vi "Configure DC Mode.vi"(0 "VISA resource name":refnum<visa-resource-name>, 1 "Voltage Low Limit (0 V)":dbl min=0.0 max=400.0 format="%.1f", 2 "Voltage High Limit (300 V)":dbl=300.0 min=0.0 max=400.0 format="%.1f", 5 "Enable Over Current Fold Back (F:Disable)":bool, 7 "Output Polarity (T:Positive)":bool=TRUE, 9 "Memory (1)":i32=1 min=1 max=50 step=1, 11 "error in (no error)":errorcluster, 12 "Output DC Voltage (115 V)":dbl=115.0 min=0.0 max=400.0 format="%.1f", 13 "Voltage Range Mode (1:Low)":u16(ring)=1 items=["High", "Low"], 14 "Current High Limit (0 A)":dbl min=0.0 max=55.2 format="%.3f") -> (4 "VISA resource name out":refnum<visa-resource-name>, 15 "error out":errorcluster)   [LabVIEW 2016, in "APT 300XAC Series.lvlib"]
doc: "Sets the instrument to DC Positive or negative mode and configures required parameters in the power source instrument.\n\nIn DC mode, the instrument can be programmed to deliver a positive DC output. A particular testing parameter setting can be configured similar to Manual Mode\n\nNote : This selection will only be available if the DC option has been installed on the AC power source."
uses:
  APT 300XAC Series.lvlib
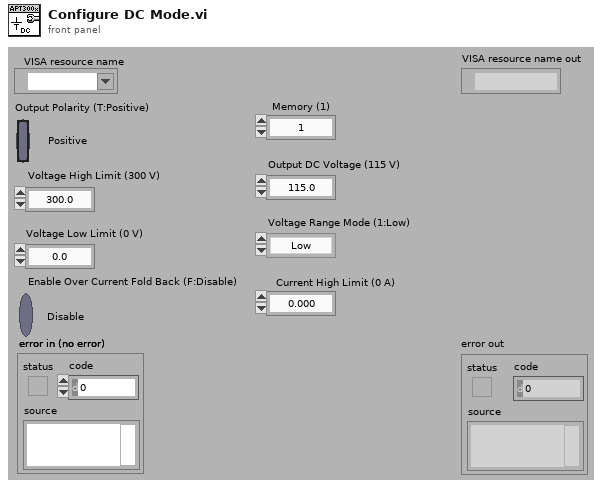
[diagram p1: front panel]
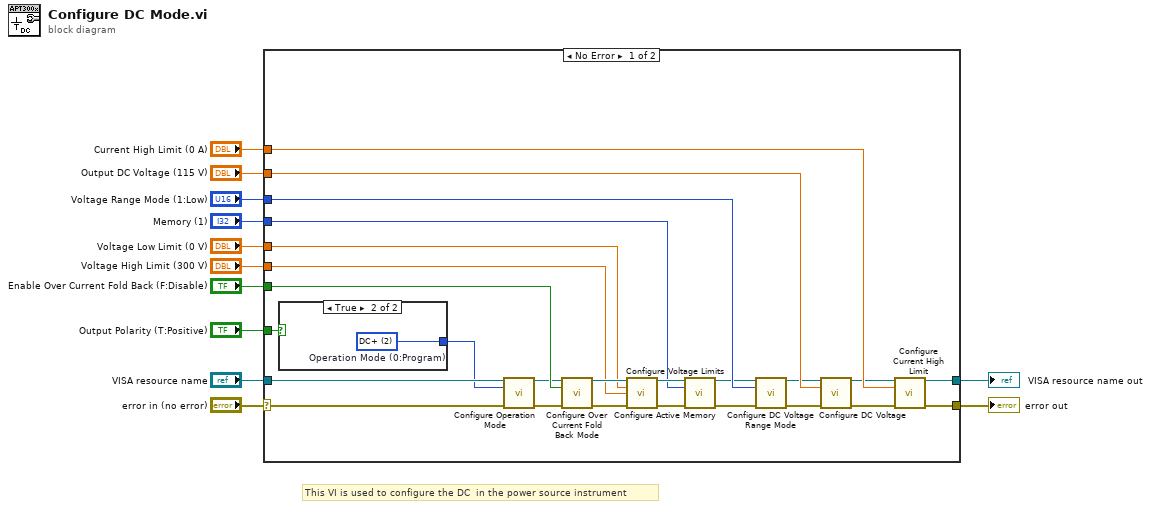
[diagram p0: block diagram]
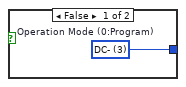
[diagram p2: hidden frame]
diagram:
  # "This VI is used to configure the DC  in the power source instrument"
  n1 = case shown="No Error" "error in (no error)" {
    selector: "error in (no error)" -> [w37 w40]
    tunnel: "VISA resource name" -> [w36 w41]
    tunnel: [w24 w41] -> w10
    tunnel: [w23 w40] -> w9
    tunnel: "Enable Over Current Fold Back (F:Disable)" -> [w35 _]
    tunnel: "Voltage Low Limit (0 V)" -> [w32 _]
    tunnel: "Voltage High Limit (300 V)" -> [w31 _]
    tunnel: "Output Polarity (T:Positive)" -> [w27 _]
    tunnel: "Current High Limit (0 A)" -> [w19 _]
    tunnel: "Voltage Range Mode (1:Low)" -> [w20 _]
    tunnel: "Output DC Voltage (115 V)" -> [w21 _]
    tunnel: "Memory (1)" -> [w22 _]
    frame No Error {
      n2 = case shown="True" w27 {
        tunnel: [w38 w39] -> w28
        frame False {
          w38 = u16 3 items=["Program", "Manual", "DC+", "DC-"]  # Operation Mode (0:Program)
        }
        frame True {
          w39 = u16 2 items=["Program", "Manual", "DC+", "DC-"]  # Operation Mode (0:Program)
        }
      }
      n3 = call "Configure Operation Mode.vi"("VISA resource name"=w36, "Operation Mode (0:Program)"=w28, "error in (no error)"=w37) -> ("VISA resource name out"=w30:refnum<visa-resource-name>, "error out"=w29:errorcluster)  [unwired: 11 in]
      n4 = call "Configure Over Current Fold Back Mode.vi"("VISA resource name"=w30, "Enable Over Current Fold Back (F:Disable)"=w35, "error in (no error)"=w29) -> ("VISA resource name out"=w34:refnum<visa-resource-name>, "error out"=w33:errorcluster)  [unwired: 11 in]
      n5 = call "Configure Voltage Limits.vi"("VISA resource name"=w34, "Voltage Low Limit (0 V)"=w32, "Voltage High Limit (300 V)"=w31, "error in (no error)"=w33) -> ("VISA resource name out"=w26:refnum<visa-resource-name>, "error out"=w25:errorcluster)  [unwired: 10 in]
      n6 = call "Configure Active Memory.vi"("VISA resource name"=w26, "Memory (1)"=w22, "error in (no error)"=w25) -> ("VISA resource name out"=w18:refnum<visa-resource-name>, "error out"=w13:errorcluster)  [unwired: 11 in]
      n7 = call "Configure DC Voltage Range Mode.vi"("VISA resource name"=w18, "Voltage Range Mode (1:Low)"=w20, "error in (no error)"=w13) -> ("VISA resource name out"=w17:refnum<visa-resource-name>, "error out"=w14:errorcluster)  [unwired: 11 in]
      n8 = call "Configure DC Voltage.vi"("VISA resource name"=w17, "Output DC Voltage (115 V)"=w21, "error in (no error)"=w14) -> ("VISA resource name out"=w16:refnum<visa-resource-name>, "error out"=w15:errorcluster)  [unwired: 11 in]
      n9 = call "Configure Current High Limit.vi"("VISA resource name"=w16, "Current High Limit (0 A)"=w19, "error in (no error)"=w15) -> ("VISA resource name out"=w24:refnum<visa-resource-name>, "error out"=w23:errorcluster)  [unwired: 11 in]
    }
    frame Error {
    }
  }
  "error out" <- w9
  "VISA resource name out" <- w10
